vi "Skyline Send Waveform Tags.vi"(8 "error in (no error)":errorcluster, 9 "Keywords":string[](array[string]), 10 "Decimate to single value":bool=TRUE, 11 "data in":waveform(dbl)[](array[waveform])) -> (0 "error out":errorcluster, 3 "data out":waveform(dbl)[](array[waveform]))   [LabVIEW 2015]
uses:
  <vilib>/TagLibrary/Data Type.ctl
  <vilib>/TagLibrary/Tag Library.lvlib
  <resource>/objmgr/niTag.rc
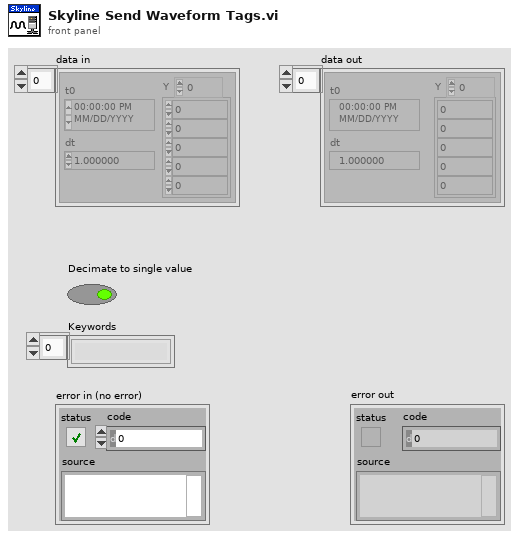
[diagram p1: front panel]
types:
  T1 = typedef "Tag Library.lvlib/Data Type.ctl" = enum32{"Double", "Int", "String"}
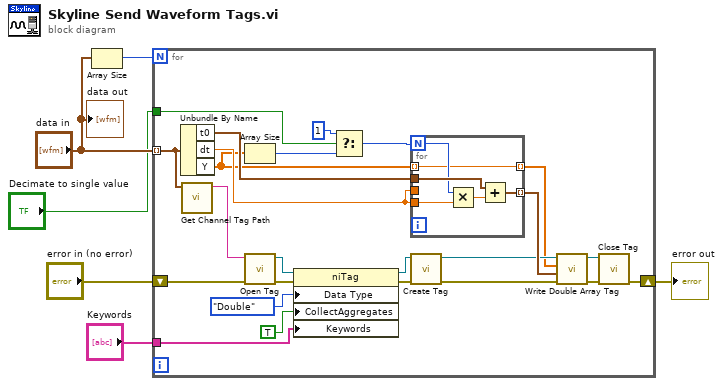
[diagram p0: block diagram]
diagram:
  n1 = Array Size(array="data in") -> (size(s)=w5:i32)
  n2 = for {
    N: w5 -> [_]
    tunnel: "data in" -> [w29] mode=indexing
    shift-right: [w24] -> w3
    shift-left: "error in (no error)" -> [w23]
    tunnel: "Decimate to single value" -> [w15]
    tunnel: "Keywords" -> [w9]
    n3 = Unbundle By Name(w29) -> ("t0"=w30:timestamp, "dt"=w21:dbl, "Y"=w10:dbl[])
    n4 = call "Get Channel Tag Path.vi"("Waveform"=w29) -> ("channel path"=w22:string)  [unwired: 10 in]
    n5 = Array Size(array=w10) -> (size(s)=w12:i32)
    n6 = call <vilib>:"Open Tag.vi"("error in (no error)"=w23, "tag path"=w22) -> ("error out"=w28:errorcluster, "tag reference (out)"=w25:refnum<k21>)  [unwired: 8 in]
    n7 = property class="niTag"(reference=w25, error in=w28, "Data Type"=Data_Type."Double", "CollectAggregates"=TRUE, "Keywords"=w9) -> (reference out=w7:refnum<k21>, error out=w8:errorcluster)
    n8 = Select(t=1, s=w15, f=w12) -> (s? t:f=w14:i32)
    n9 = for {
      N: w14 -> [w34]
      tunnel: w30 -> [w36]
      tunnel: w21 -> [_]
      tunnel: w21 -> [w33]
      tunnel: [w32] -> w20 mode=indexing
      tunnel: [w31] -> w11 mode=indexing
      tunnel: w10 -> [w31] mode=indexing
      n10 = Multiply(x=w34, y=w33) -> (x*y=w35:dbl)
      n11 = Add(x=w36, y=w35) -> (x+y=w32:timestamp)
    }
    n12 = call <vilib>:"Create Tag.vi"("error in (no error)"=w8, "tag reference (in)"=w7) -> ("error out"=w17:errorcluster, "tag reference (out)"=w19:refnum<k21>)  [unwired: 8 in]
    n13 = call <vilib>:"Write Double Array Tag.vi"("error in (no error)"=w17, "timestamps"=w20, "doubles"=w11, "tag reference (in)"=w19) -> ("error out"=w16:errorcluster, "tag reference (out)"=w18:refnum<k21>)  [unwired: 6 in]
    n14 = call <vilib>:"Close Tag.vi"("error in (no error)"=w16, "tag reference (in)"=w18) -> ("error out"=w24:errorcluster)  [unwired: 9 in]
  }
  "error out" <- w3
  "data out" <- "data in"
